vi "Snap to Baseline.vi"(8 "Starting Line Y":dbl format="%#_13g", 9 "Snap to baseline":bool, 10 "Point in":cluster{"x":dbl, "y":dbl, "th":dbl}, 11 "Picture in":refnum<vi>) -> (3 "Point out":cluster{"x":dbl, "y":dbl, "th":dbl})   [LabVIEW 2023]
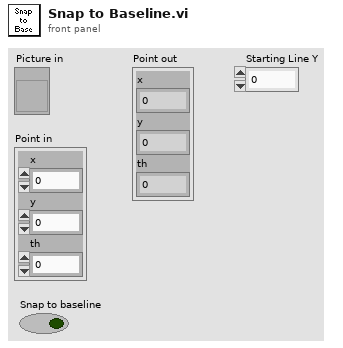
[diagram p1: front panel]
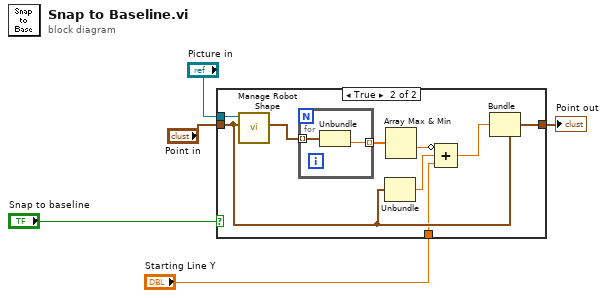
[diagram p0: block diagram]
diagram:
  n1 = case shown="True" "Snap to baseline" {
    tunnel: "Point in" -> [w6 w9]
    tunnel: [w6 w8] -> w4
    tunnel: "Picture in" -> [_ w13]
    tunnel: "Starting Line Y" -> [_ w7]
    frame False {
    }
    frame True {
      n2 = call "Manage Robot Shape.vi"("Robot Position (ft)"=w9, "Pict Ref"=w13) -> ("Boundary Poly"=w15:cluster{dbl, dbl}[])  [unwired: 7 in, 2 out]
      n3 = for {
        tunnel: w15 -> [w17] mode=indexing
        tunnel: [w16] -> w14 mode=indexing
        n4 = Unbundle(w17) -> (w16:dbl)  [unwired: 1 out]
      }
      n5 = Unbundle(w9) -> ("y"=w11:dbl)  [unwired: 2 out]
      n6 = Array Max & Min(array=w14) -> (min value=w12:dbl)  [unwired: 3 out]
      n7 = Compound Arithmetic op=ADD(invert w12, w11, w7) -> (w10:dbl)
      n8 = Bundle(cluster=w9, "y"=w10) -> (w8:cluster{"x":dbl, "y":dbl, "th":dbl})  [unwired: 2 in]
    }
  }
  "Point out" <- w4
